vi "Flipper Control Servo.vi"(2 "Frisbee States":T1, 3 "Cannon Position(deg)":dbl, 4 "Enable Stack":bool, 5 "override flipper":bool) -> (0 "Stop Conveyer Belt":bool, 1 "Set Flipper's Servos Angle":i32)   [LabVIEW 2012]
panel:
  # "Flipper Angle"
  # "Cannon Angle"
  # "90"
  # "90-min / 90"
  # "170"
  # "0 / min angle"
  # "90 / min+90"
  # "48.6 => 49"
  # "-min angle / 0"
  # "0"
  # "original angle / \"Cannon Position(deg)\""
  # "FlipperAtPlace is True if the servo is at 0 degrees"
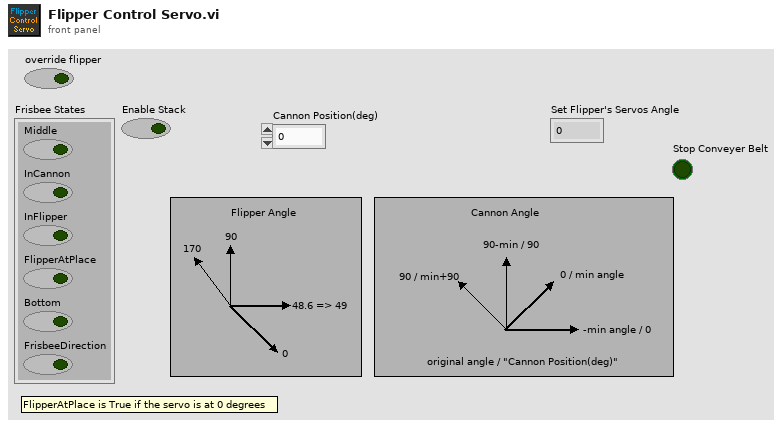
[diagram p1: front panel]
types:
  T1 = cluster{"Middle":bool, "InCannon":bool, "InFlipper":bool, "FlipperAtPlace":bool, "Bottom":bool, "FrisbeeDirection":bool}
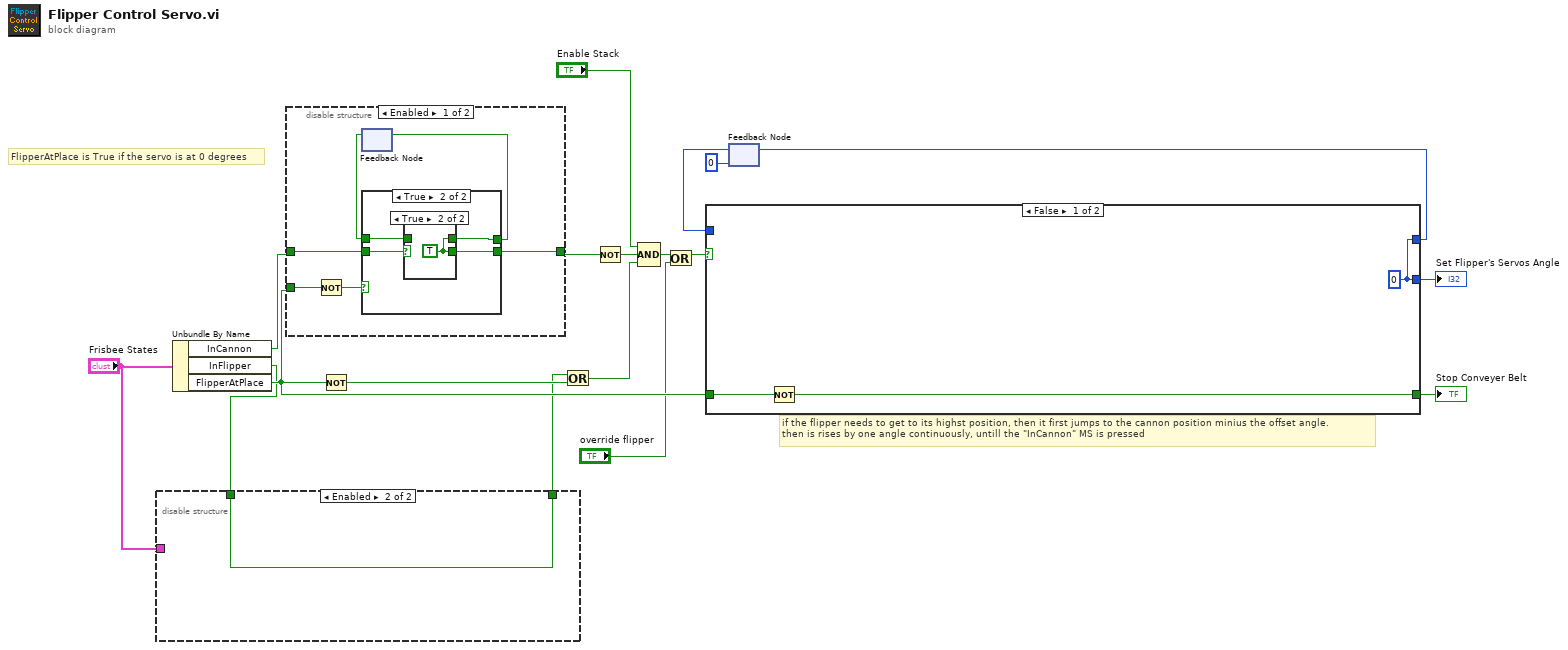
[diagram p0: block diagram]
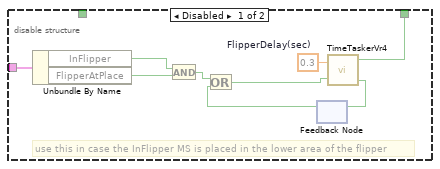
[diagram p2: hidden frame]
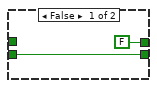
[diagram p3: hidden frame]
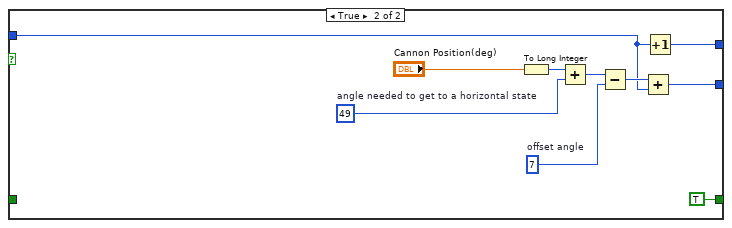
[diagram p6: hidden frame]
diagram:
  # "FlipperAtPlace is True if the servo is at 0 degrees"
  # "if the flipper needs to get to its highst position, then it first jumps to the cannon position minius the offset angle.\nthen is rises by one angle continuously, untill the \"InCannon\" MS is pressed"
  n1 = Unbundle By Name("Frisbee States") -> ("InCannon"=w7:bool, "InFlipper"=w4:bool, "FlipperAtPlace"=w8:bool)
  n2 = disable-structure shown="Enabled" {
    disable-tunnel: "Frisbee States" -> [w27 _]
    disable-tunnel: [w19 w28] -> w3
    disable-tunnel: w4 -> [_ w28]
    frame Disabled {
      w20 = 0.3  # FlipperDelay(sec)
      # "use this in case the InFlipper MS is placed in the lower area of the flipper"
      n3 = Unbundle By Name(w27) -> ("InFlipper"=w22:bool, "FlipperAtPlace"=w21:bool)
      n4 = And(x=w22, y=w21) -> (x .and. y?=w26:bool)
      n5 = feedback #1() -> (w25:bool)  [unwired: 1 in]
      n6 = Or(x=w26, y=w25) -> (x .or. y?=w23:bool)
      n7 = call "TimeTaskerVr4.vi"("Delay(sec)"=w20, "Start Counting?"=w23) -> ("TimePast?"=w19:bool, "Counting?"=w24:bool)  [unwired: 1 out]
      n8 = feedback-in #1(w24) -> ()
    }
    frame Enabled {
    }
  }
  n9 = disable-structure shown="Enabled" {
    disable-tunnel: w8 -> [w31 _]
    disable-tunnel: w7 -> [w30 w43]
    disable-tunnel: [w29 w43] -> w6
    frame Enabled {
      n10 = Not(x=w31) -> (.not. x?=w32:bool)
      n11 = feedback #2() -> (w33:bool)  [unwired: 1 in]
      n12 = case shown="True" w32 {
        tunnel: [w36 w37] -> w29
        tunnel: w30 -> [w36 w40]
        tunnel: [FALSE w39] -> w34
        tunnel: w33 -> [_ w38]
        frame False {
        }
        frame True {
          n13 = case shown="True" w40 {
            tunnel: [w41 w42] -> w39
            tunnel: w38 -> [w41 _]
            tunnel: [w41 w42] -> w37
            frame False {
            }
            frame True {
              w42 = TRUE
            }
          }
        }
      }
      n14 = feedback-in #2(w34) -> ()
    }
    frame Disabled {
      # "use this in case the InCannon MS is\nplaced on the flipper at all time"
    }
  }
  n15 = Not(x=w8) -> (.not. x?=w16:bool)
  n16 = Or(x=w3, y=w16) -> (x .or. y?=w17:bool)
  n17 = Not(x=w6) -> (.not. x?=w18:bool)
  n18 = Compound Arithmetic op=AND("Enable Stack", w18, w17) -> (w15:bool)
  n19 = Or(x=w15, y="override flipper") -> (x .or. y?=w2:bool)
  n20 = feedback #3(0) -> (w13:i32)
  n21 = case shown="False" w2 {
    tunnel: [w46 w50] -> w12
    tunnel: [w46 w51] -> w14
    tunnel: w13 -> [_ w49]
    tunnel: [w44 TRUE ("Stop Conveyer Belt")] -> w10
    tunnel: w8 -> [w45 _]
    frame False {
      w46 = 0
      n22 = Not(x=w45) -> (.not. x?=w44:bool)
    }
    frame True {
      w56 = 49  # angle needed to get to a horizontal state
      w54 = 7  # offset angle
      n23 = To Long Integer(number="Cannon Position(deg)") -> (32bit integer=w53:i32)
      n24 = Add(x=w53, y=w56) -> (x+y=w55:i32)
      n25 = Subtract(x=w55, y=w54) -> (x-y=w52:i32)
      n26 = Add(x=w52, y=w49) -> (x+y=w50:i32)
      n27 = Increment(x=w49) -> (x+1=w51:i32)
    }
  }
  "Set Flipper's Servos Angle" <- w12
  "Stop Conveyer Belt" <- w10
  n28 = feedback-in #3(w14) -> ()
